vi "Clear.vi"(8 "error in (no error)":errorcluster, 11 "VISA resource name":refnum<visa-resource-name>) -> (0 "error out":errorcluster, 3 "VISA resource name out":refnum<visa-resource-name>)   [LabVIEW 2020, in "QuPMXdriver.lvlib"]
doc: "Resets the instrument and then sends a set of default setup commands to the instrument.\nAll the slaves are opened (signal relays turned OFF and GND relays turned ON). Error bits on status byte are cleared."
uses:
  QuPMXdriver.lvlib
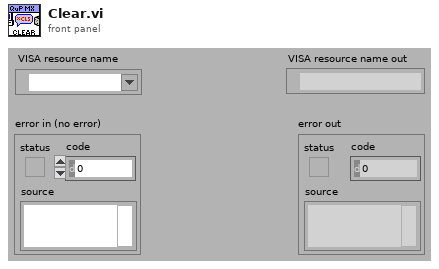
[diagram p1: front panel]
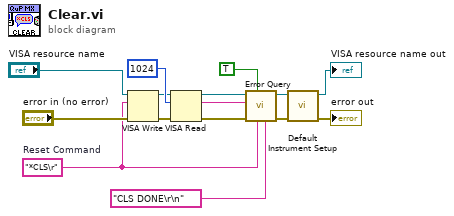
[diagram p0: block diagram]
diagram:
  w3 = "*CLS\r"  # Reset Command
  n1 = VISA Write(VISA resource name="VISA resource name", write buffer=w3, error in (no error)="error in (no error)") -> (VISA resource name out=w11:refnum<visa-resource-name>, error out=w1:errorcluster)  [unwired: 1 out]
  n2 = VISA Read(VISA resource name=w11, byte count=u32 1024, error in (no error)=w1) -> (VISA resource name out=w9:refnum<visa-resource-name>, read buffer=w4:string, error out=w10:errorcluster)  [unwired: 1 out]
  n3 = call "Error Query.vi"("Expected read buffer"="CLS DONE\r\n" ("Correct answer"), "Last command"=w3, "Ignore empty sequence? (T)"=TRUE ("Ignore empty sequence?"), "error in (no error)"=w10, "Read buffer"=w4, "VISA resource name"=w9) -> ("error out"=w8:errorcluster, "VISA resource name out"=w5:refnum<visa-resource-name>)  [unwired: 4 in]
  n4 = call "Default Instrument Setup.vi"("error in (no error)"=w8, "VISA resource name"=w5) -> ("error out"=→"error out":errorcluster, "VISA resource name out"=→"VISA resource name out":refnum<visa-resource-name>)  [unwired: 8 in]
